vi "Create.vi"(5 "Collection Is Equivalent in":refnum<class "Collection Is Equivalent.lvclass">, 8 "error in (no error)":errorcluster, 11 "Other":variant) -> (0 "error out":errorcluster, 3 "Collection Is Equivalent":refnum<class "Collection Is Equivalent.lvclass">)   [LabVIEW 2017, in "Transparent Assertions.lvlib" / "Constraints.lvlib" / "Collection Is Equivalent.lvclass"]
uses:
  Collection Is Equivalent.lvclass
  Collection Is Equivalent.lvclass/Collection Is Equivalent.ctl
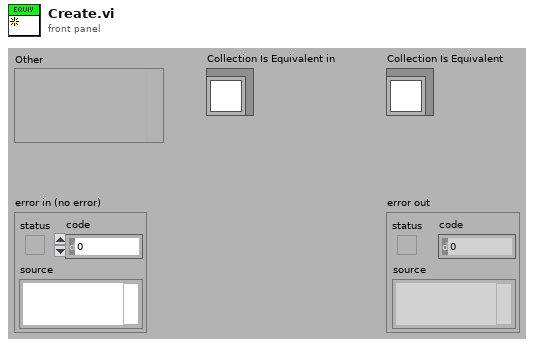
[diagram p1: front panel]
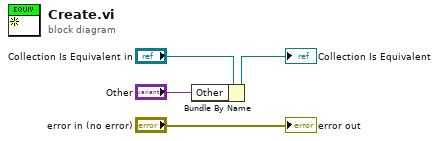
[diagram p0: block diagram]
diagram:
  n1 = Bundle By Name(cluster="Collection Is Equivalent in", "Other"="Other") -> (→"Collection Is Equivalent":refnum<class "Collection Is Equivalent.lvclass">)
  "error out" <- "error in (no error)"
